vi "Get Log Waveforms.vi"(7 "RT Data in":T1={"Device Ref"=18446744073709551615, "Waveforms"=[], "Channels"={"Command Chan Refs"=[], "Command Data Refs"=[], "Command Values"=[], "Status Chan Refs"=[], "Status Data Refs"=[], "Status Values"=[], "System Time"={"System Time"=timestamp(0 s since 1904-01-01), "Data Reference"=0, "Absolute Time Channel Data Ref"=0, "Get Date-Time Channel Data Ref"=0}, "Trigger Chan Refs"=[], "Trigger Data Refs"=[], "Trigger Values"=[]}, "Waveform Logs"=[], "Communication"={"Async Status"=refnum, "Wfm Comm Properties"={"WPL"={"Custom Queue Size"=1, "Use Custom Queue Size?"=FALSE}}, "Shutdown Event"=refnum, "Trigger Event"=refnum, "New File Event"=refnum, "Log Queues"=[], "Async VI Ref"=refnum}, "error"={"status"=FALSE, "code"=0, "source"=""}} {"Device Ref" format="%.0x"; "Channels"."Trigger Data Refs"."Data Reference" format="%.0x"; "Channels"."Trigger Chan Refs" format="%.0x"; "Channels"."System Time"."Get Date-Time Channel Data Ref" format="%.0x"; "Channels"."System Time"."Absolute Time Channel Data Ref" format="%.0x"; "Channels"."System Time"."Channel Data Reference" format="%.0x"; "Channels"."Status Data Refs"."Data Reference" format="%.0x"; "Channels"."Command Data Refs"."Data Reference" format="%.0x"; "Channels"."Status Chan Refs" format="%.0x"; "Channels"."Command Chan Refs" format="%.0x"; "Waveforms"."Waveform Ref in" format="%.0x"; "Waveform Logs"."Node ID" format="%.0x"; "Waveform Logs"."TDMS Error Code"."Data Ref" format="%.0x"; "Waveform Logs"."Missed Samples"."Data Ref" format="%.0x"; "Waveform Logs"."File Status"."Data Ref" format="%.0x"; "Waveform Logs"."Start New File"."Data Ref" format="%.0x"; "Waveform Logs"."Logging Enabled"."Data Ref" format="%.0x"; "Waveform Logs"."Stop Trigger"."Node Data Ref" format="%.0x"; "Waveform Logs"."Stop Trigger"."Node ID" format="%.0x"; "Waveform Logs"."Start Trigger"."Node Data Ref" format="%.0x"; "Waveform Logs"."Start Trigger"."Node ID" format="%.0x"}, 11 "Log Index in":i32, 12 "Version year":string) -> (8 "RT Data out":T1={"Device Ref"=18446744073709551615, "Waveforms"=[], "Channels"={"Command Chan Refs"=[], "Command Data Refs"=[], "Command Values"=[], "Status Chan Refs"=[], "Status Data Refs"=[], "Status Values"=[], "System Time"={"System Time"=timestamp(0 s since 1904-01-01), "Data Reference"=0, "Absolute Time Channel Data Ref"=0, "Get Date-Time Channel Data Ref"=0}, "Trigger Chan Refs"=[], "Trigger Data Refs"=[], "Trigger Values"=[]}, "Waveform Logs"=[], "Communication"={"Async Status"=refnum, "Wfm Comm Properties"={"WPL"={"Custom Queue Size"=1, "Use Custom Queue Size?"=FALSE}}, "Shutdown Event"=refnum, "Trigger Event"=refnum, "New File Event"=refnum, "Log Queues"=[], "Async VI Ref"=refnum}, "error"={"status"=FALSE, "code"=0, "source"=""}} {"Device Ref" format="%.0x"; "Channels"."Trigger Data Refs"."Data Reference" format="%.0x"; "Channels"."Trigger Chan Refs" format="%.0x"; "Channels"."System Time"."Get Date-Time Channel Data Ref" format="%.0x"; "Channels"."System Time"."Absolute Time Channel Data Ref" format="%.0x"; "Channels"."System Time"."Channel Data Reference" format="%.0x"; "Channels"."Status Data Refs"."Data Reference" format="%.0x"; "Channels"."Command Data Refs"."Data Reference" format="%.0x"; "Channels"."Status Chan Refs" format="%.0x"; "Channels"."Command Chan Refs" format="%.0x"; "Waveforms"."Waveform Ref in" format="%.0x"; "Waveform Logs"."Node ID" format="%.0x"; "Waveform Logs"."TDMS Error Code"."Data Ref" format="%.0x"; "Waveform Logs"."Missed Samples"."Data Ref" format="%.0x"; "Waveform Logs"."File Status"."Data Ref" format="%.0x"; "Waveform Logs"."Start New File"."Data Ref" format="%.0x"; "Waveform Logs"."Logging Enabled"."Data Ref" format="%.0x"; "Waveform Logs"."Stop Trigger"."Node Data Ref" format="%.0x"; "Waveform Logs"."Stop Trigger"."Node ID" format="%.0x"; "Waveform Logs"."Start Trigger"."Node Data Ref" format="%.0x"; "Waveform Logs"."Start Trigger"."Node ID" format="%.0x"}, 15 "Log Index out":i32)   [LabVIEW 2015, in "Waveform Data Logger Engine.lvlib"]
uses:
  Waveform Data Logger Engine.lvlib
  Types/RT Data.ctl
  <vilib>/NI Veristand/Custom Device API/Custom Device Item Ref.ctl
  Types/Inline Waveform Info.ctl
  <vilib>/NI Veristand/Custom Device API/Waveform Data Reference.ctl
  Classes/Waveforms/Waveform Receive/Associated Log.ctl
  <vilib>/NI Veristand/Custom Device API/Custom Device Waveform DataType.ctl
  Types/Channels.ctl
  <vilib>/NI Veristand/Custom Device API/Block Data Reference.ctl
  <vilib>/NI Veristand/Custom Device API/Data Reference.ctl
  Types/System Time.ctl
  Types/Inline Waveform Log Info.ctl
  Shared/Classes/Log File Specifications/Waveform TDMS Log File Specification/Waveform TDMS Log File Specification.lvclass
  Classes/Triggers/Trigger/Trigger.lvclass
  Types/Inline Log Waveform.ctl
  Types/Trigger Settings.ctl
  Types/Log Status.ctl
  Types/Channel.ctl
  Types/Communication.ctl
  Types/Async Status.ctl
  Types/Async State.ctl
  <vilib>/NI Veristand/Custom Device Waveform API/Communication Properties.ctl
  Types/Trigger Event Data.ctl
  Types/Trigger Received.ctl
  Types/New File Event Data.ctl
  Types/Log Queues.ctl
  Shared/Globals/Property Strings.vi
  <vilib>/NI Veristand/Custom Device API/Get Item Property (String Array).vi
  <vilib>/NI Veristand/Custom Device API/Get Item Property (U32 Array).vi
  <vilib>/NI VeriStand/Custom Device Tools/Custom Device Utility Library/Custom Device Utility Library.lvlib
  Shared/Waveform Data Logger Shared.lvlib
  <vilib>/NI VeriStand/Custom Device API/Custom Device API.lvlib
  Classes/Waveforms/Waveform Receive/Waveform Receive.lvclass
  <vilib>/NI Veristand/Custom Device Waveform API/NI_VS Custom Device Waveform API.lvlib
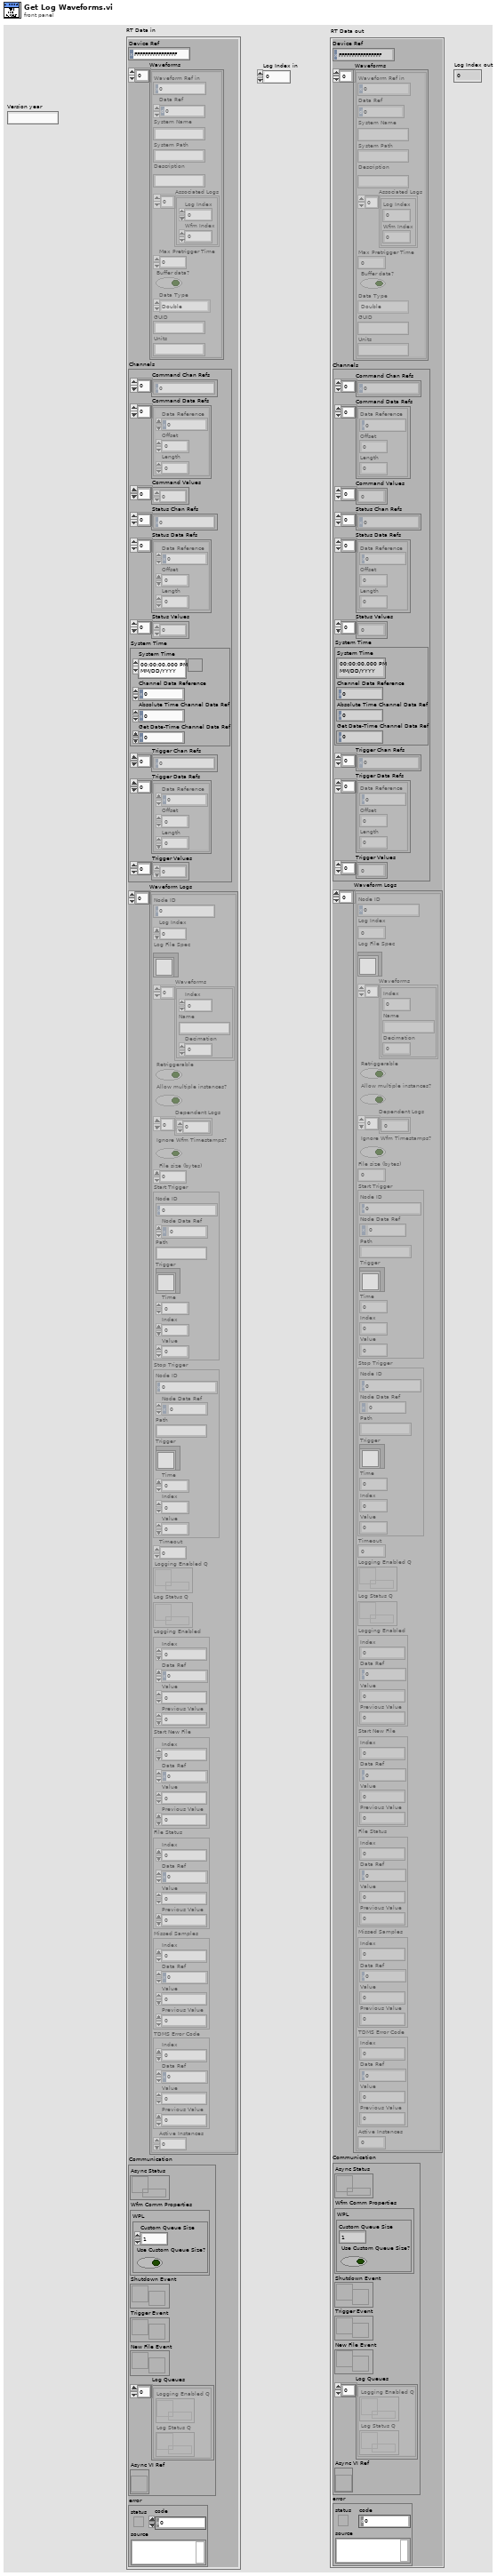
[diagram p1: front panel]
types:
  T1 = typedef "Waveform Data Logger Engine.lvlib/RT Data.ctl" = cluster{"Device Ref":T2, "Waveforms":T3[], "Channels":T7, "Waveform Logs":T11[], "Communication":T15, "error":errorcluster}
  T2 = typedef "Custom Device API.lvlib/Custom Device Item Ref.ctl" = u64
  T3 = typedef "Waveform Data Logger Engine.lvlib/Inline Waveform Info.ctl" = cluster{"Waveform Ref in":T2, "Data Ref":T4, "System Name":string, "System Path":string, "Description":string, "Associated Logs":T5[], "Max Pretrigger Time":dbl, "Buffer data?":bool, "Data Type":T6, "GUID":string, "Units":string}
  T4 = typedef "Custom Device API.lvlib/Waveform Data Reference.ctl" = i32
  T5 = typedef "Waveform Data Logger Engine.lvlib/Waveform Receive.lvclass/Associated Log.ctl" = cluster{"Log Index":i32, "Wfm Index":i32}
  T6 = typedef "Custom Device API.lvlib/Custom Device Waveform DataType.ctl" = enum16{"Double", "Complex Double"}
  T7 = typedef "Waveform Data Logger Engine.lvlib/Channels.ctl" = cluster{"Command Chan Refs":T2[], "Command Data Refs":T8[], "Command Values":dbl[], "Status Chan Refs":T2[], "Status Data Refs":T8[], "Status Values":dbl[], "System Time":T10, "Trigger Chan Refs":T2[], "Trigger Data Refs":T8[], "Trigger Values":dbl[]}
  T8 = typedef "Custom Device API.lvlib/Block Data Reference.ctl" = cluster{"Data Reference":T9, "Offset":u64, "Length":u64}
  T9 = typedef "Custom Device API.lvlib/Data Reference.ctl" = i32
  T10 = typedef "Waveform Data Logger Engine.lvlib/System Time.ctl" = cluster{"System Time":timestamp, "Data Reference":T9, "Absolute Time Channel Data Ref":T9, "Get Date-Time Channel Data Ref":T9}
  T11 = typedef "Waveform Data Logger Engine.lvlib/Inline Waveform Log Info.ctl" = cluster{"Node ID":T2, "Log Index":i32, "Log File Spec":refnum<class "Waveform TDMS Log File Specification.lvclass">, "Waveforms":T12[], "Retriggerable":bool, "Allow multiple instances?":bool, "Dependent Logs":i32[], "Ignore Wfm Timestamps?":bool, "File size (bytes)":i64, "Start Trigger":T13, "Stop Trigger":T13, "Timeout":dbl, "Logging Enabled Q":refnum<queue>, "Log Status Q":refnum<queue>, "Logging Enabled":T14, "Start New File":T14, "File Status":T14, "Missed Samples":T14, "TDMS Error Code":T14, "Active Instances":i32}
  T12 = typedef "Waveform Data Logger Engine.lvlib/Inline Log Waveform.ctl" = cluster{"Index":i32, "Name":string, "Decimation":u32}
  T13 = typedef "Waveform Data Logger Engine.lvlib/Trigger Settings.ctl" = cluster{"Node ID":T2, "Node Data Ref":i32, "Path":string, "Trigger":refnum<class "Trigger.lvclass">, "Time":dbl, "Index":i32, "Value":dbl}
  T14 = typedef "Waveform Data Logger Engine.lvlib/Channel.ctl" = cluster{"Index":i32, "Data Ref":T9, "Value":dbl, "Previous Value":dbl}
  T15 = typedef "Waveform Data Logger Engine.lvlib/Communication.ctl" = cluster{"Async Status":refnum<queue>, "Wfm Comm Properties":T16, "Shutdown Event":refnum<user-event>, "Trigger Event":refnum<user-event>, "New File Event":refnum<user-event>, "Log Queues":T17[], "Async VI Ref":refnum<vi>}
  T16 = typedef "NI_VS Custom Device Waveform API.lvlib/Communication Properties.ctl" = cluster{"WPL":cluster{"Custom Queue Size":i32, "Use Custom Queue Size?":bool}}
  T17 = typedef "Waveform Data Logger Engine.lvlib/Log Queues.ctl" = cluster{"Logging Enabled Q":refnum<queue>, "Log Status Q":refnum<queue>}
  T18 = typedef "Custom Device API.lvlib/Custom Device Waveform.ctl" = cluster{"Data Type":T6, "Units":string}
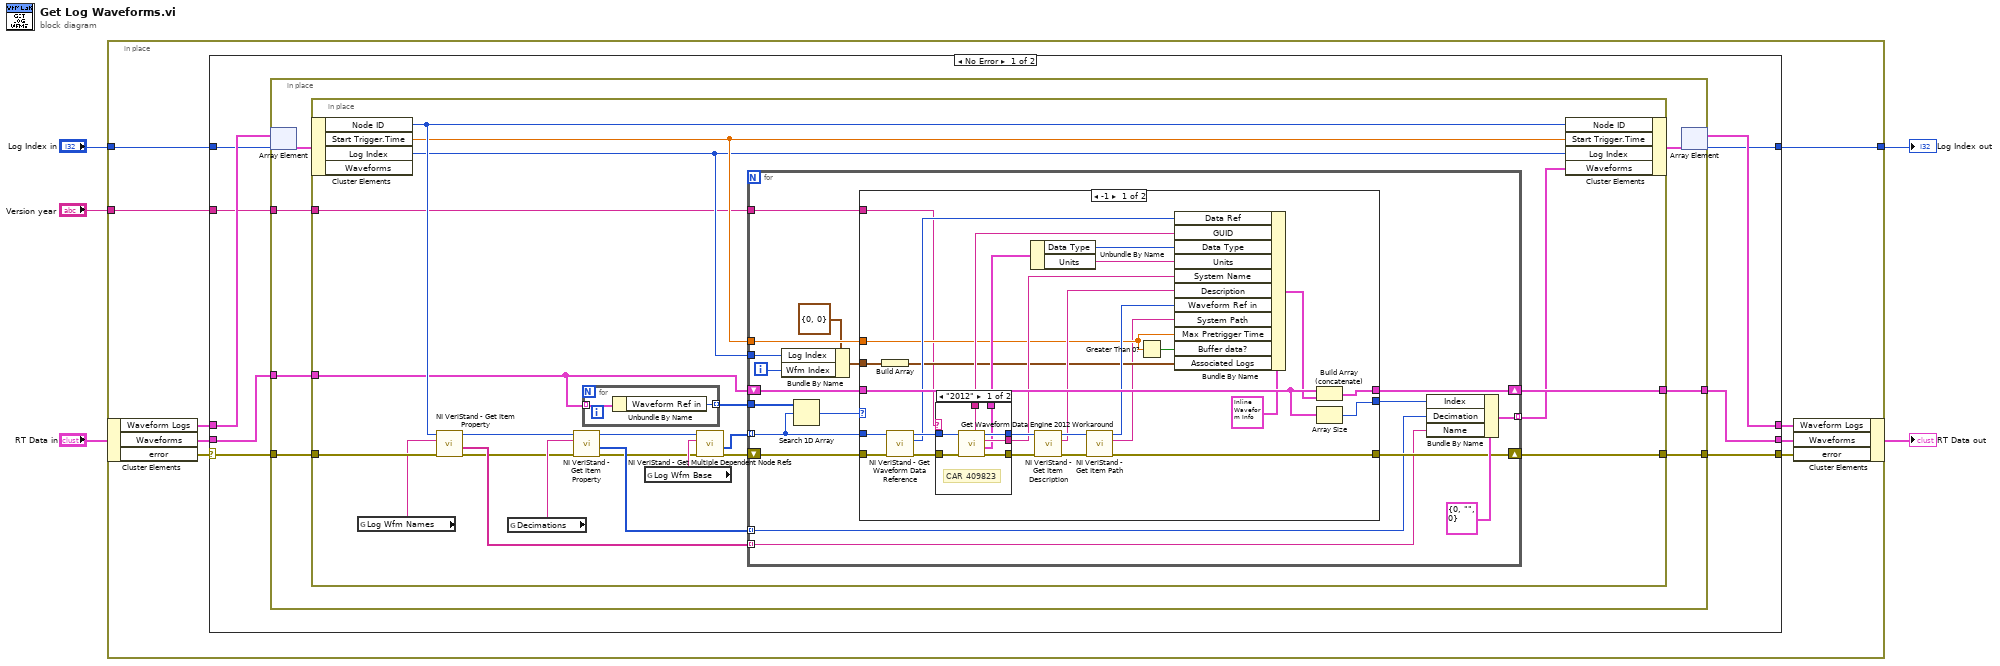
[diagram p0: block diagram]
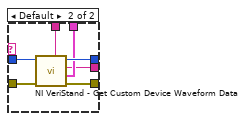
[diagram p2: hidden frame]
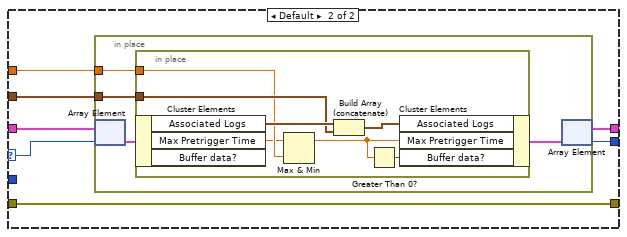
[diagram p3: hidden frame]
diagram:
  n1 = in-place {
    in-place-border: "Log Index in" -> [w10]
    in-place-border: [w8] -> w2
    in-place-border: "Version year" -> [w6]
    n2 = in-place-cluster #1("RT Data in") -> ("Waveform Logs"=w11:T11[], "Waveforms"=w14:T3[], "error"=w7:errorcluster)
    n3 = case shown="No Error" w7 {
      selector: w7 -> [w16 w132]
      tunnel: w14 -> [w23 w133]
      tunnel: [w22 w133] -> w13
      tunnel: [w21 w132] -> w12
      tunnel: w11 -> [w20 w134]
      tunnel: w10 -> [w19 w135]
      tunnel: [w18 w134] -> w9
      tunnel: [w17 w135] -> w8
      tunnel: w6 -> [w15 _]
      frame No Error {
        n4 = in-place {
          in-place-border: w16 -> [w30]
          in-place-border: w23 -> [w29]
          in-place-border: [w28] -> w22
          in-place-border: [w27] -> w21
          in-place-border: w15 -> [w24]
          n5 = in-place-array #2(w20, w19) -> (w26:T11)
          n6 = in-place {
            in-place-border: w30 -> [w51]
            in-place-border: w29 -> [w32]
            in-place-border: [w50] -> w28
            in-place-border: [w49] -> w27
            in-place-border: w24 -> [w31]
            n7 = in-place-cluster #3(w26) -> ("Node ID"=w35:T2, "Start Trigger.Time"=w34:dbl, "Log Index"=w33:i32)  [unwired: 1 out]
            n8 = global read "Property Strings.vi" "Log Wfm Names"() -> (w47:string)
            n9 = call-poly <vilib>:"NI VeriStand - Get Item Property.vi"("error in (no error)"=w51, "Property Name"=w47, "Item Ref in"=w35) -> ("error out"=w41:errorcluster, "Value"=w43:string[], "Item Ref out"=w40:T2)  [unwired: 1 in, 5 out]
            n10 = global read "Property Strings.vi" "Decimations"() -> (w48:string)
            n11 = call-poly <vilib>:"NI VeriStand - Get Item Property.vi"("error in (no error)"=w41, "Property Name"=w48, "Item Ref in"=w40) -> ("error out"=w38:errorcluster, "Value"=w42:u32[], "Item Ref out"=w39:T2)  [unwired: 1 in, 5 out]
            n12 = for {
              tunnel: w32 -> [w53] mode=indexing
              tunnel: [w52] -> w45 mode=indexing
              n13 = Unbundle By Name(w53) -> ("Waveform Ref in"=w52:T2)
            }
            n14 = global read "Property Strings.vi" "Log Wfm Base"() -> (w46:string)
            n15 = call <vilib>:"NI VeriStand - Get Multiple Dependent Node Refs.vi"("error in (no error)"=w38, "Base Property Name"=w46, "Item Ref in"=w39) -> ("error out"=w37:errorcluster, "Dependent Node Refs"=w44:T2[])  [unwired: 6 in, 1 out]
            n16 = for {
              shift-right: [w69] -> w50
              shift-left: w32 -> [w70]
              tunnel: w45 -> [w68]
              tunnel: w44 -> [w67] mode=indexing
              tunnel: w43 -> [w55] mode=indexing
              tunnel: w42 -> [w56] mode=indexing
              tunnel: [w65] -> w36 mode=indexing
              shift-right: [w63] -> w49
              shift-left: w37 -> [w64]
              tunnel: w34 -> [w61]
              tunnel: w33 -> [w59]
              tunnel: w31 -> [w54]
              i -> [w58]
              n17 = Bundle By Name(cluster=T5 {"Log Index"=0, "Wfm Index"=0} ("Associated Log"), "Log Index"=w59, "Wfm Index"=w58) -> (w57:T5)
              n18 = Search 1D Array(1D array=w68, element=w67) -> (index of element=w71:i32)  [unwired: 1 in]
              n19 = case shown="-1" w71 {
                selector: w71 -> [_ w119]
                tunnel: [w98 w118] -> w62
                tunnel: w70 -> [w99 w120]
                tunnel: [w97 w117] -> w69
                tunnel: w67 -> [w74 _]
                tunnel: w64 -> [w90 w116]
                tunnel: [w73 w116] -> w63
                tunnel: w61 -> [w78 w115]
                tunnel: w57 -> [w81 w114]
                tunnel: w54 -> [w72 _]
                frame -1 {
                  n20 = Build Array(w81) -> (w80:T5[])
                  n21 = call <vilib>:"NI VeriStand - Get Waveform Data Reference.vi"("error in (no error)"=w90, "Waveform Ref in"=w74) -> ("error out"=w95:errorcluster, "Waveform Data Reference"=w89:T4, "Waveform Ref out"=w96:T2)  [unwired: 7 in]
                  n22 = case shown="\"2012\"" w72 {
                    tunnel: w96 -> [w100 w113]
                    tunnel: w95 -> [w106 w112]
                    tunnel: [w103 w111] -> w94
                    tunnel: [w105 w110] -> w91
                    tunnel: [w101 w109] -> w88
                    tunnel: [w102 w108] -> w85
                    tunnel: [w104 w107] -> w84
                    frame "2012" {
                      # "CAR 409823"
                      n23 = call "Get Waveform Data Engine 2012 Workaround.vi"("error in (no error)"=w106, "Waveform Ref in"=w100) -> ("error out"=w105:errorcluster, "Waveform"=w102:T18, "Waveform Name"=w104:string, "Waveform Ref out"=w103:T2, "GUID"=w101:string)  [unwired: 4 in, 1 out]
                    }
                    frame Default {
                      n24 = call <vilib>:"NI VeriStand - Get Custom Device Waveform Data.vi"("error in (no error)"=w112, "Waveform Ref in"=w113) -> ("error out"=w110:errorcluster, "Waveform"=w108:T18, "Waveform Name"=w107:string, "Waveform Ref out"=w111:T2, "GUID"=w109:string)  [unwired: 4 in, 1 out]
                    }
                  }
                  n25 = Unbundle By Name(w85) -> ("Data Type"=w87:T6, "Units"=w86:string)
                  n26 = call <vilib>:"NI VeriStand - Get Item Description.vi"("error in (no error)"=w91, "Item Ref in"=w94) -> ("error out"=w92:errorcluster, "Description"=w83:string, "Item Ref out"=w93:T2)  [unwired: 6 in, 1 out]
                  n27 = call <vilib>:"NI VeriStand - Get Item Path.vi"("error in (no error)"=w92, "Item Ref in"=w93) -> ("error out"=w73:errorcluster, "Path"=w75:string, "Item Ref out"=w82:T2)  [unwired: 6 in, 1 out]
                  n28 = Greater Than 0?(x=w78) -> (x > 0?=w79:bool)
                  n29 = Bundle By Name(cluster=T3 {"Waveform Ref in"=0, "Data Ref"=0, "System Name"="", "System Path"="", "Description"="", "Associated Logs"=[], "Max Pretrigger Time"=0.0, "Buffer data?"=FALSE, "Data Type"=enum."Double", "GUID"="", "Units"=""} ("Inline Waveform Info"), "Data Ref"=w89, "GUID"=w88, "Data Type"=w87, "Units"=w86, "System Name"=w84, "Description"=w83, "Waveform Ref in"=w82, "System Path"=w75, "Max Pretrigger Time"=w78, "Buffer data?"=w79, "Associated Logs"=w80) -> (w77:T3)
                  n30 = Build Array (concatenate)(w99, w77) -> (w97:T3[])
                  n31 = Array Size(array=w99) -> (size(s)=w98:i32)
                }
                frame Default {
                  n32 = in-place {
                    in-place-border: w114 -> [w123]
                    in-place-border: w115 -> [w122]
                    n33 = in-place-array #4(w120, w119) -> (w124:T3)
                    n34 = in-place {
                      in-place-border: w123 -> [w130]
                      in-place-border: w122 -> [w129]
                      n35 = in-place-cluster #5(w124) -> ("Associated Logs"=w131:T5[], "Max Pretrigger Time"=w128:dbl)  [unwired: 1 out]
                      n36 = Max & Min(x=w128, y=w129) -> (max(x,y)=w125:dbl)  [unwired: 1 out]
                      n37 = Build Array (concatenate)(w131, w130) -> (w127:T5[])
                      n38 = Greater Than 0?(x=w125) -> (x > 0?=w126:bool)
                      n39 = in-place-cluster #5("Associated Logs"=w127, "Max Pretrigger Time"=w125, "Buffer data?"=w126) -> (w121:T3)
                    }
                    n40 = in-place-array #4(w121) -> (w117:T3[], w118:i32)
                  }
                }
              }
              n41 = Bundle By Name(cluster=T12 {"Index"=0, "Name"="", "Decimation"=0} ("Inline Log Waveform"), "Index"=w62, "Decimation"=w56, "Name"=w55) -> (w65:T12)
            }
            n42 = in-place-cluster #3("Node ID"=w35, "Start Trigger.Time"=w34, "Log Index"=w33, "Waveforms"=w36) -> (w25:T11)
          }
          n43 = in-place-array #2(w25) -> (w18:T11[], w17:i32)
        }
      }
      frame Error {
      }
    }
    n44 = in-place-cluster #1("Waveform Logs"=w9, "Waveforms"=w13, "error"=w12) -> (→"RT Data out":T1)
  }
  "Log Index out" <- w2
